vi "Create Run.vi"(0 "Sift Client in":refnum<class "Sift Client.lvclass">, 5 "Name":string, 7 "Description":string, 9 "Tags":string[](array[string]), 11 "error in (no error)":errorcluster) -> (4 "Sift Client out":refnum<class "Sift Client.lvclass">, 6 "Run ID":string, 15 "error out":errorcluster)   [LabVIEW 2024, in "Sift Client.lvlib" / "Sift Client.lvclass"]
doc: "Create a Sift Run.\n\nSee https://docs.siftstack.com/docs/data-model/assets-channels-runs#runs for more details."
uses:
  Sift Client.lvclass
  Private/Typedefs/Messages/JSON Request.ctl
  Private/Typedefs/Messages/Create Run Request.ctl
  Private/Typedefs/Messages/Create Run Response.ctl
  Sift Client.lvclass/Sift Client.ctl
  <vilib>/addons/_JKI.lib/Serialization/JSON/JKI JSON Serialization.lvlib
  Sift Client.lvlib
panel:
  in  "Create Run Response":T1
  in  "Create Run Request":T2
  in  "JSON Request":T3
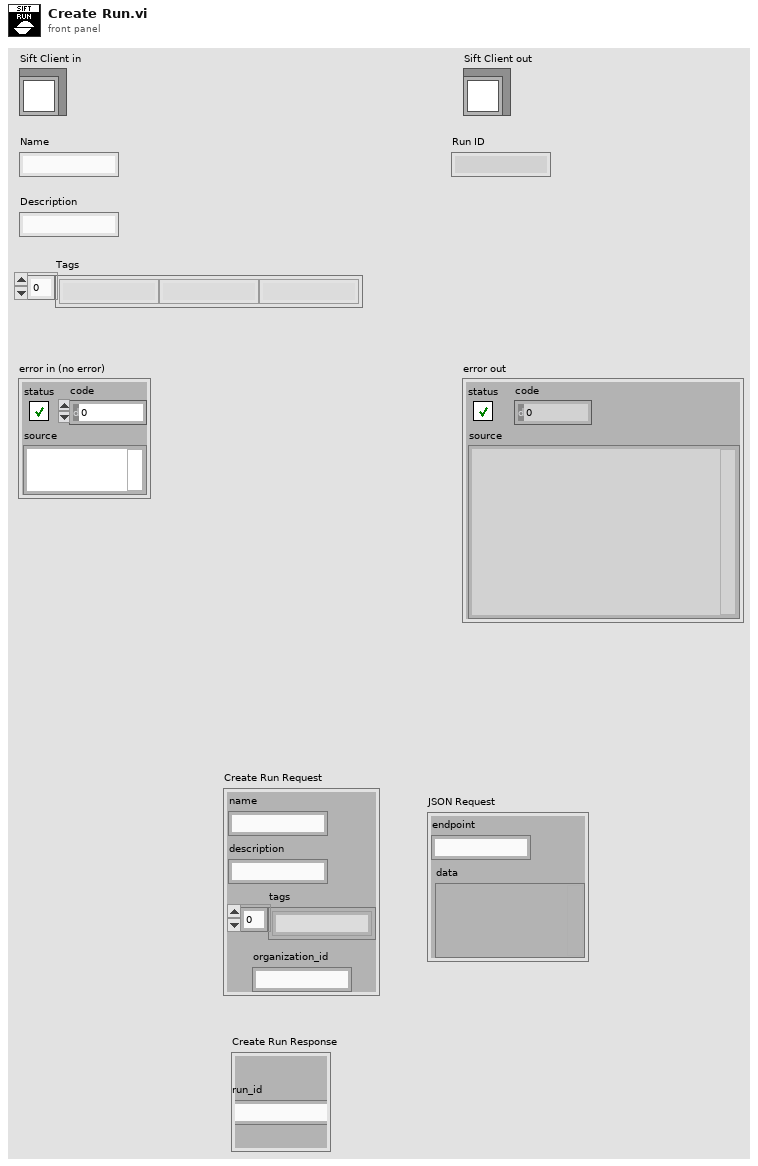
[diagram p1: front panel]
types:
  T1 = typedef "Sift Client.lvlib/Create Run Response.ctl" = cluster{"run_id":string}
  T2 = typedef "Sift Client.lvlib/Create Run Request.ctl" = cluster{"name":string, "description":string, "tags":string[], "organization_id":string}
  T3 = typedef "Sift Client.lvlib/JSON Request.ctl" = cluster{"endpoint":string, "data":variant}
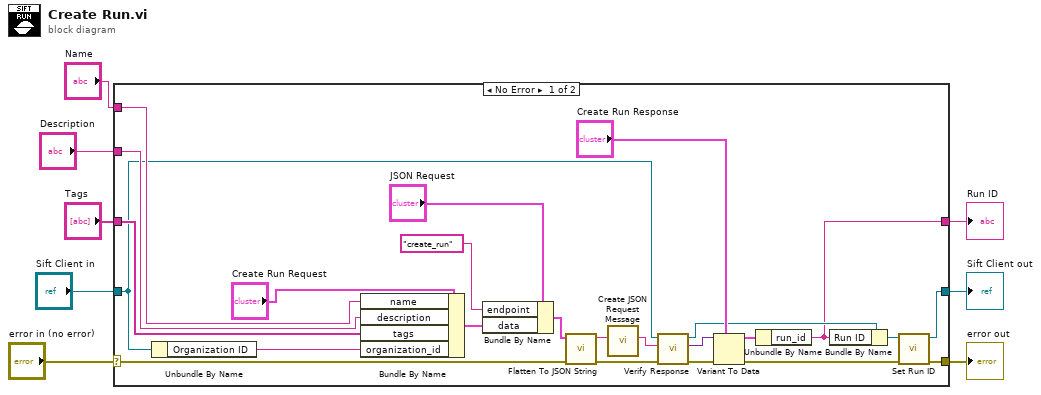
[diagram p0: block diagram]
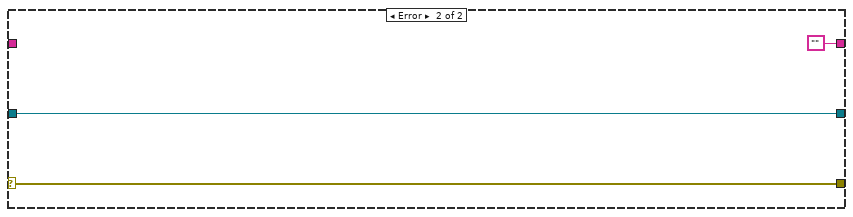
[diagram p2: hidden frame]
diagram:
  n1 = case shown="No Error" "error in (no error)" {
    selector: "error in (no error)" -> [w15 w35]
    tunnel: [w9 w35] -> w7
    tunnel: [w11 w33] -> w6
    tunnel: "Name" -> [w30 _]
    tunnel: "Description" -> [w29 _]
    tunnel: "Tags" -> [w28 _]
    tunnel: [w17 ""] -> w2
    tunnel: "Sift Client in" -> [w22 w33]
    frame No Error {
      n2 = Unbundle By Name(w22) -> ("Organization ID"=w27:string)
      n3 = Bundle By Name(cluster="Create Run Request", "name"=w30, "description"=w29, "tags"=w28, "organization_id"=w27) -> (w26:T2)
      n4 = Bundle By Name(cluster="JSON Request", "endpoint"="create_run", "data"=w26) -> (w25:T3)
      n5 = call <vilib>:"Flatten To JSON String.vi"("error in"=w15, "Variant"=w25) -> ("error out"=w14:errorcluster, "JSON String"=w24:string)  [unwired: 8 in]
      n6 = call "Create JSON Request Message.vi"("Data"=w24) -> ("Message"=w23:string)  [unwired: 10 in]
      n7 = call-dynamic "Verify Response.vi"("error in (no error)"=w14, "Message"=w23, "Sift Client in"=w22) -> ("error out"=w13:errorcluster, "data"=w21:variant, "Sift Client out"=w18:refnum<class "Sift Client.lvclass">)  [unwired: 6 in]
      n8 = Variant To Data(error in=w13, type="Create Run Response", Variant=w21) -> (data=w19:T1, error out=w10:errorcluster)
      n9 = Unbundle By Name(w19) -> ("run_id"=w17:string)
      n10 = Bundle By Name(cluster=w18, "Run ID"=w17) -> (w12:refnum<class "Sift Client.lvclass">)
      n11 = call-dynamic "Set Run ID.vi"("error in (no error)"=w10, "Sift Client in"=w12) -> ("error out"=w9:errorcluster, "Sift Client out"=w11:refnum<class "Sift Client.lvclass">)  [unwired: 8 in]
    }
    frame Error {
    }
  }
  "error out" <- w7
  "Sift Client out" <- w6
  "Run ID" <- w2
